vi "main 0.4.vi"() -> ()   [LabVIEW 2015]
uses:
  subvi/PHOIBOS/DEFINITIONS/DEF_dev_state.ctl
  subvi/PHOIBOS/DEFINITIONS/DEF_dev_type.ctl
  <vilib>/Utility/file.llb/Write Delimited Spreadsheet (DBL).vi
  subvi/Newport ESP301/Newport ESP301.lvlib
  subvi/sp_manip.llb/sp_manip_lib.lvlib
  subvi/sp_manip.llb/tcp_gateway.lvlib
panel:
  out "state":T1 items=["Off"=-1, "Standby"=0, "On"=1]
  in  "BasePath 2":path=path "Z:/PESdata"
  out "ESP_con?":bool caption="ESP301"
  out "phoib_con?":bool caption="PHOIBOS"
  out "manip_con?":bool caption="manipulator"
  out "cam_con?":bool caption="camera"
  in  "main_close":bool
  in  "Tab Control":enum32{"Live", "Measure", "Settings", "Devices"}(tab)
  in  "cam_dark#":u32 max=1000
  in  "cam_dark":bool
  out "cam_fps":dbl(slide)=8.239338102188393 caption="FPS" scale=0.1..50.0
  out "cam_burst_progress":u8(slide) scale=0.0..200.0
  in  "cam_burstnr":u32 max=1000
  in  "cam_burst":bool
  in  "ESP_delta":dbl
  in  "ESP_+ 2":bool
  in  "ESP_+":bool
  in  "ESP_go":bool
  in  "ESP_dest_t":dbl caption="Delay"
  in  "ESP_dest":dbl caption="Position"
  in  "ESP_set_t0":bool
  in  "phoib_I_6s":dbl=3200.0
  in  "phoib_I_5s":dbl=1400.0
  in  "phoib_I_4s":dbl=4.2
  in  "phoib_I_3s":dbl
  in  "phoib_I_2s":dbl=35.0
  in  "phoib_I_1s":dbl=21.9
  in  "phoib_standby":bool
  in  "phoib_set":bool
  out "phoib_I_6":dbl caption="Screen Voltage"
  out "phoib_I_5":dbl caption="Detctor Voltage"
  out "phoib_I_4":dbl caption="Work Function"
  out "phoib_I_3":dbl caption="Coil Current"
  out "phoib_I_2":dbl caption="Pass Energy"
  out "phoib_I_1":dbl caption="Kinetic Energy"
  out "CCD temp [°C]":i32=-12
  out "electronics temp [°C]":i32=30
  out "Saved Positions":string[][](table)=[["ertwertwert", "-2.299945", "-2.030214", "38.900024", "50.000762", "0.000887", "-97.998082"], ["uztgugt", "-14.999451", "-13.638894", "442.380066", "13.998380", "-1.893758", "-76.305838"], ["asdf", "-14.999451", "-13.638894", "442.380066", "13.998380", "-1.893758", "-76.305838"], ["test3", "-14.999451", "-13.638894", "441.380066", "13.998380", "-1.893758", "-76.305838"]]
  in  "Save Pos":bool
  in  "Load":bool
  in  "Delete":bool
  in  "ManipRel":dbl=1.0
  in  "ManipRel +":bool
  in  "ManipRel -":bool
  in  "manip.rel.select":enum32{"x", "y", "z", "polar", "tilt", "azimut"}(radio)=enum."polar"
  in  "Move Abs":bool
  in  "stop manip":bool
  in  "dest":dbl[](array[numeric])=[0.007141549166819264, -0.009888298846365134, 431.30615234375, 89.00040512814502, 1.109125024699864, -227.9162918846475] caption="destinations" format="%#.5g"
  out "names":string[](array[string])=["x", "y", "z", "polar", "tilt", "azimut"]
  out "pos":dbl[](array[numeric])=[0.007141549166819264, -0.009888298846365134, 431.30615234375, 89.00040512814502, 1.109125024699864, -227.9162918846475] caption="positions" format="%.5f"
  out "Intensity Graph":dbl[][](graph)
  in  "Exposure [ms]":u32=20
  in  "Mode":T2(ring)=enum."WideAngleMode"
  in  "VoltageRange":enum16{"3.5kV", "1.5kV", "400V", "100V", "10V"}(ring)=enum."400V"
  out "ESP_pos":dbl caption="Position"
  out "ESP_delay":dbl caption="Delay"
  in  "ESP_t0":dbl caption="Time Zero @"
  in  "binning":u16(ring)=2 items=["X 1", "X 2", "X 4", "X 8"]
  in  "Gain":bool
  out "max value":u16=55
  out "phoib_I_7":dbl caption="Conversion Voltage"
  in  "phoib_I_7s":dbl
  in  "phoib_I_8s":dbl
  in  "phoib_I_9s":dbl
  out "phoib_I_8":dbl caption="FD1"
  out "phoib_I_9":dbl caption="FD2"
  in  "cam_dark?":bool caption="subtract dark?"
  out "opti_frames":dbl=25.0 caption="#steps_opti"
  out "opti_current_frame":i32=25
  out "Measurement Progress":u8(slide) scale=0.0..100.0
  out "Camera Aquisition":u8(slide) scale=0.0..100.0
  in  "Optimize":bool
  in  "OptiStepSize":dbl=-1.0 caption="Step Size"
  in  "OptiRange":dbl=25.0 caption="Range"
  in  "meas_axis":string(combo)="tilt" caption="Axis"
  in  "meas_avg":i32=60 caption="Frames2Average"
  in  "OptiCancel":bool
  out "#steps_opti":dbl=25.0
  out "current_step_opti":i32=25
  out "ETA":string
  in  "BasePath":path=path "Z:/PESdata"
  in  "Path":path=path "Z:/software/ManipulatorControl/save.txt"
  in  "ROI Bottom":i32=32
  in  "ROI Top":i32=1
  in  "ROI Right":i32=40
  in  "ROI Left":i32=1
  in  "ESP Axis":i32=1 min=1 max=3
  in  "manip_init":bool
  in  "manip_release":bool
  in  "phoib_init":bool
  in  "phoib_release":bool
  in  "ESP_init":bool
  in  "ESP_release":bool
  in  "ESP301 VISA":refnum<visa-resource-name>="COM8"
  in  "cam_boardnr":i32
  in  "cam_init":bool
  in  "cam_release":bool
  out "error out":errorcluster
  out "error out 2":errorcluster
  # "step _ of _"
  # "step _ of _"
  # "manip"
  # "phoib"
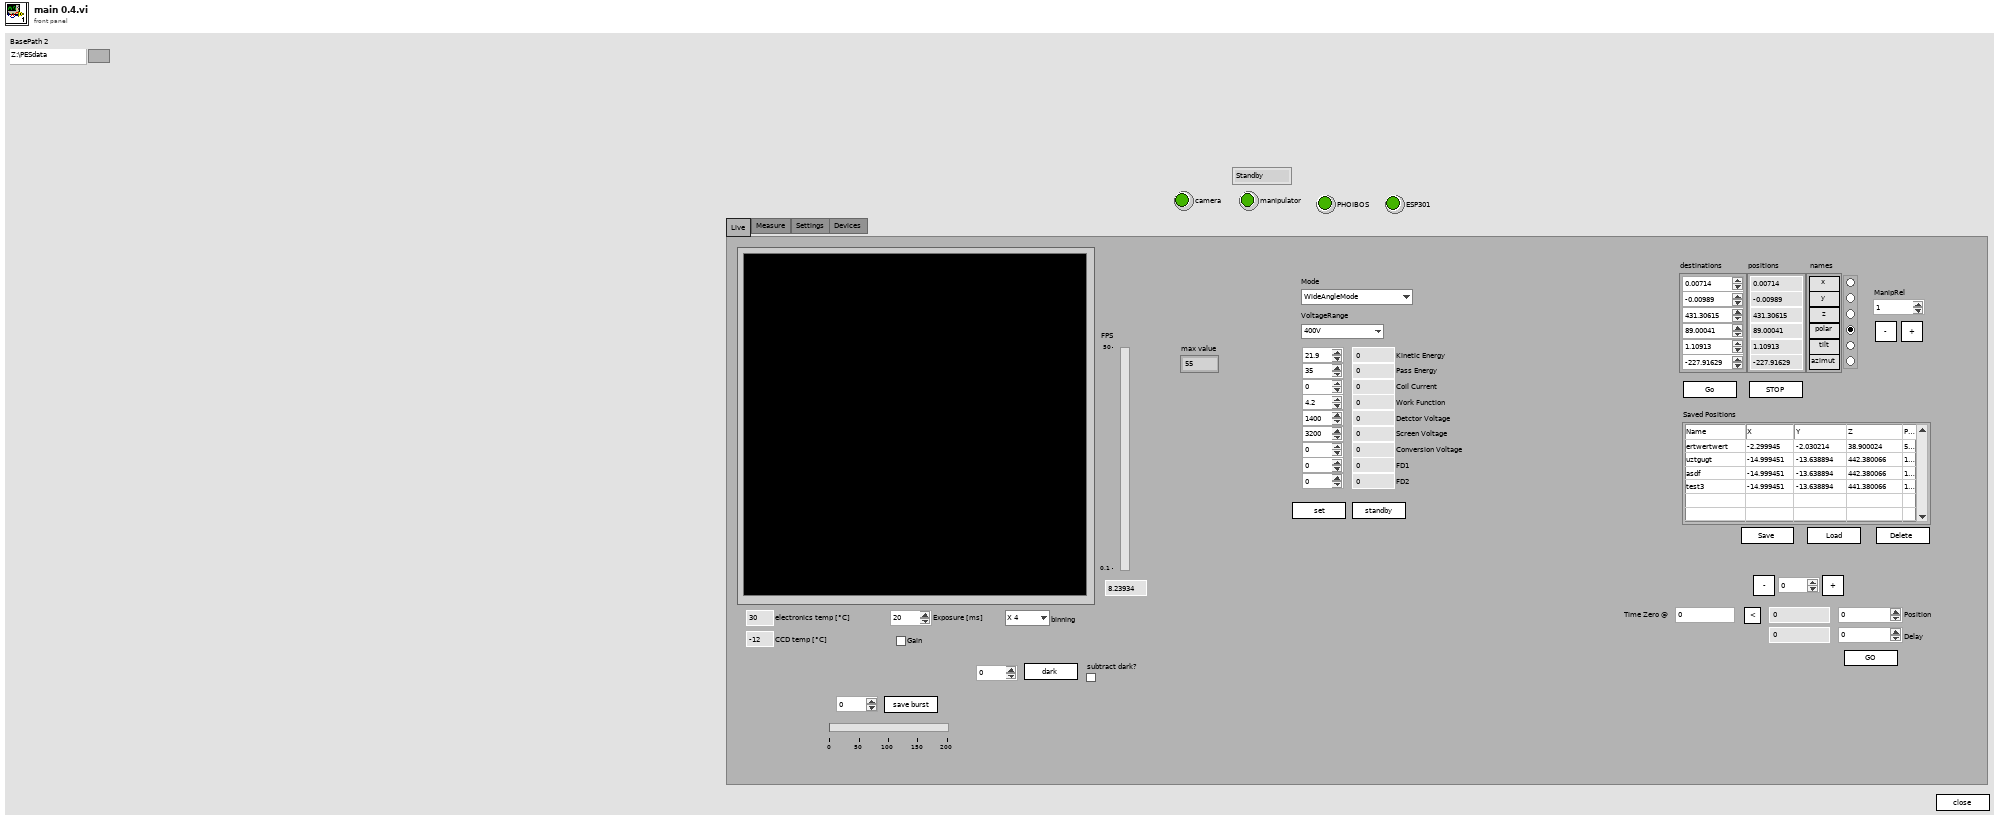
[diagram p1: front panel]
types:
  T1 = typedef "DEF_dev_state.ctl" = i32
  T2 = enum16{"HighMagnification", "MediumMagnification", "LowMagnification", "HighAngularDispersion", "MediumAngularDispersion", "LowAngularDispersion", "WideAngleMode", "LargeArea", "MediumArea", "SmallArea", "HighMagnification2", "SmallArea2", "ImagingMode"}
  T3 = cluster{"Camera type":u32, "Operating mode\nHP & QE / HS & DiCam Pro ":u32, "Frame trigger \n(High Performance and QE only)":u16, "Sequence trigger":u16, "Low Light\n(QE only)":bool, "Gain":bool, "Horzontal\nbinning":u16, "Vertical\nbinning ":u16, "ROI Left":i32, "ROI Right":i32, "ROI Top":i32, "ROI Bottom":i32}
  T4 = enum16{"open", "replace", "create", "open or create", "replace or create", "replace or create with confirmation"}
  T5 = cluster{"Axis_Name":string, "Axis_Type":string, "Axis_Position":dbl, "continous":bool, "moving":bool}[]
  T6 = cluster{"Axis_Name":string, "Axis_Type":string, "Axis_Position":dbl, "continous":bool, "moving":bool}
  T7 = typedef "DEF_dev_type.ctl" = enum32{"devA (analyzer)", "devD (detector)"}
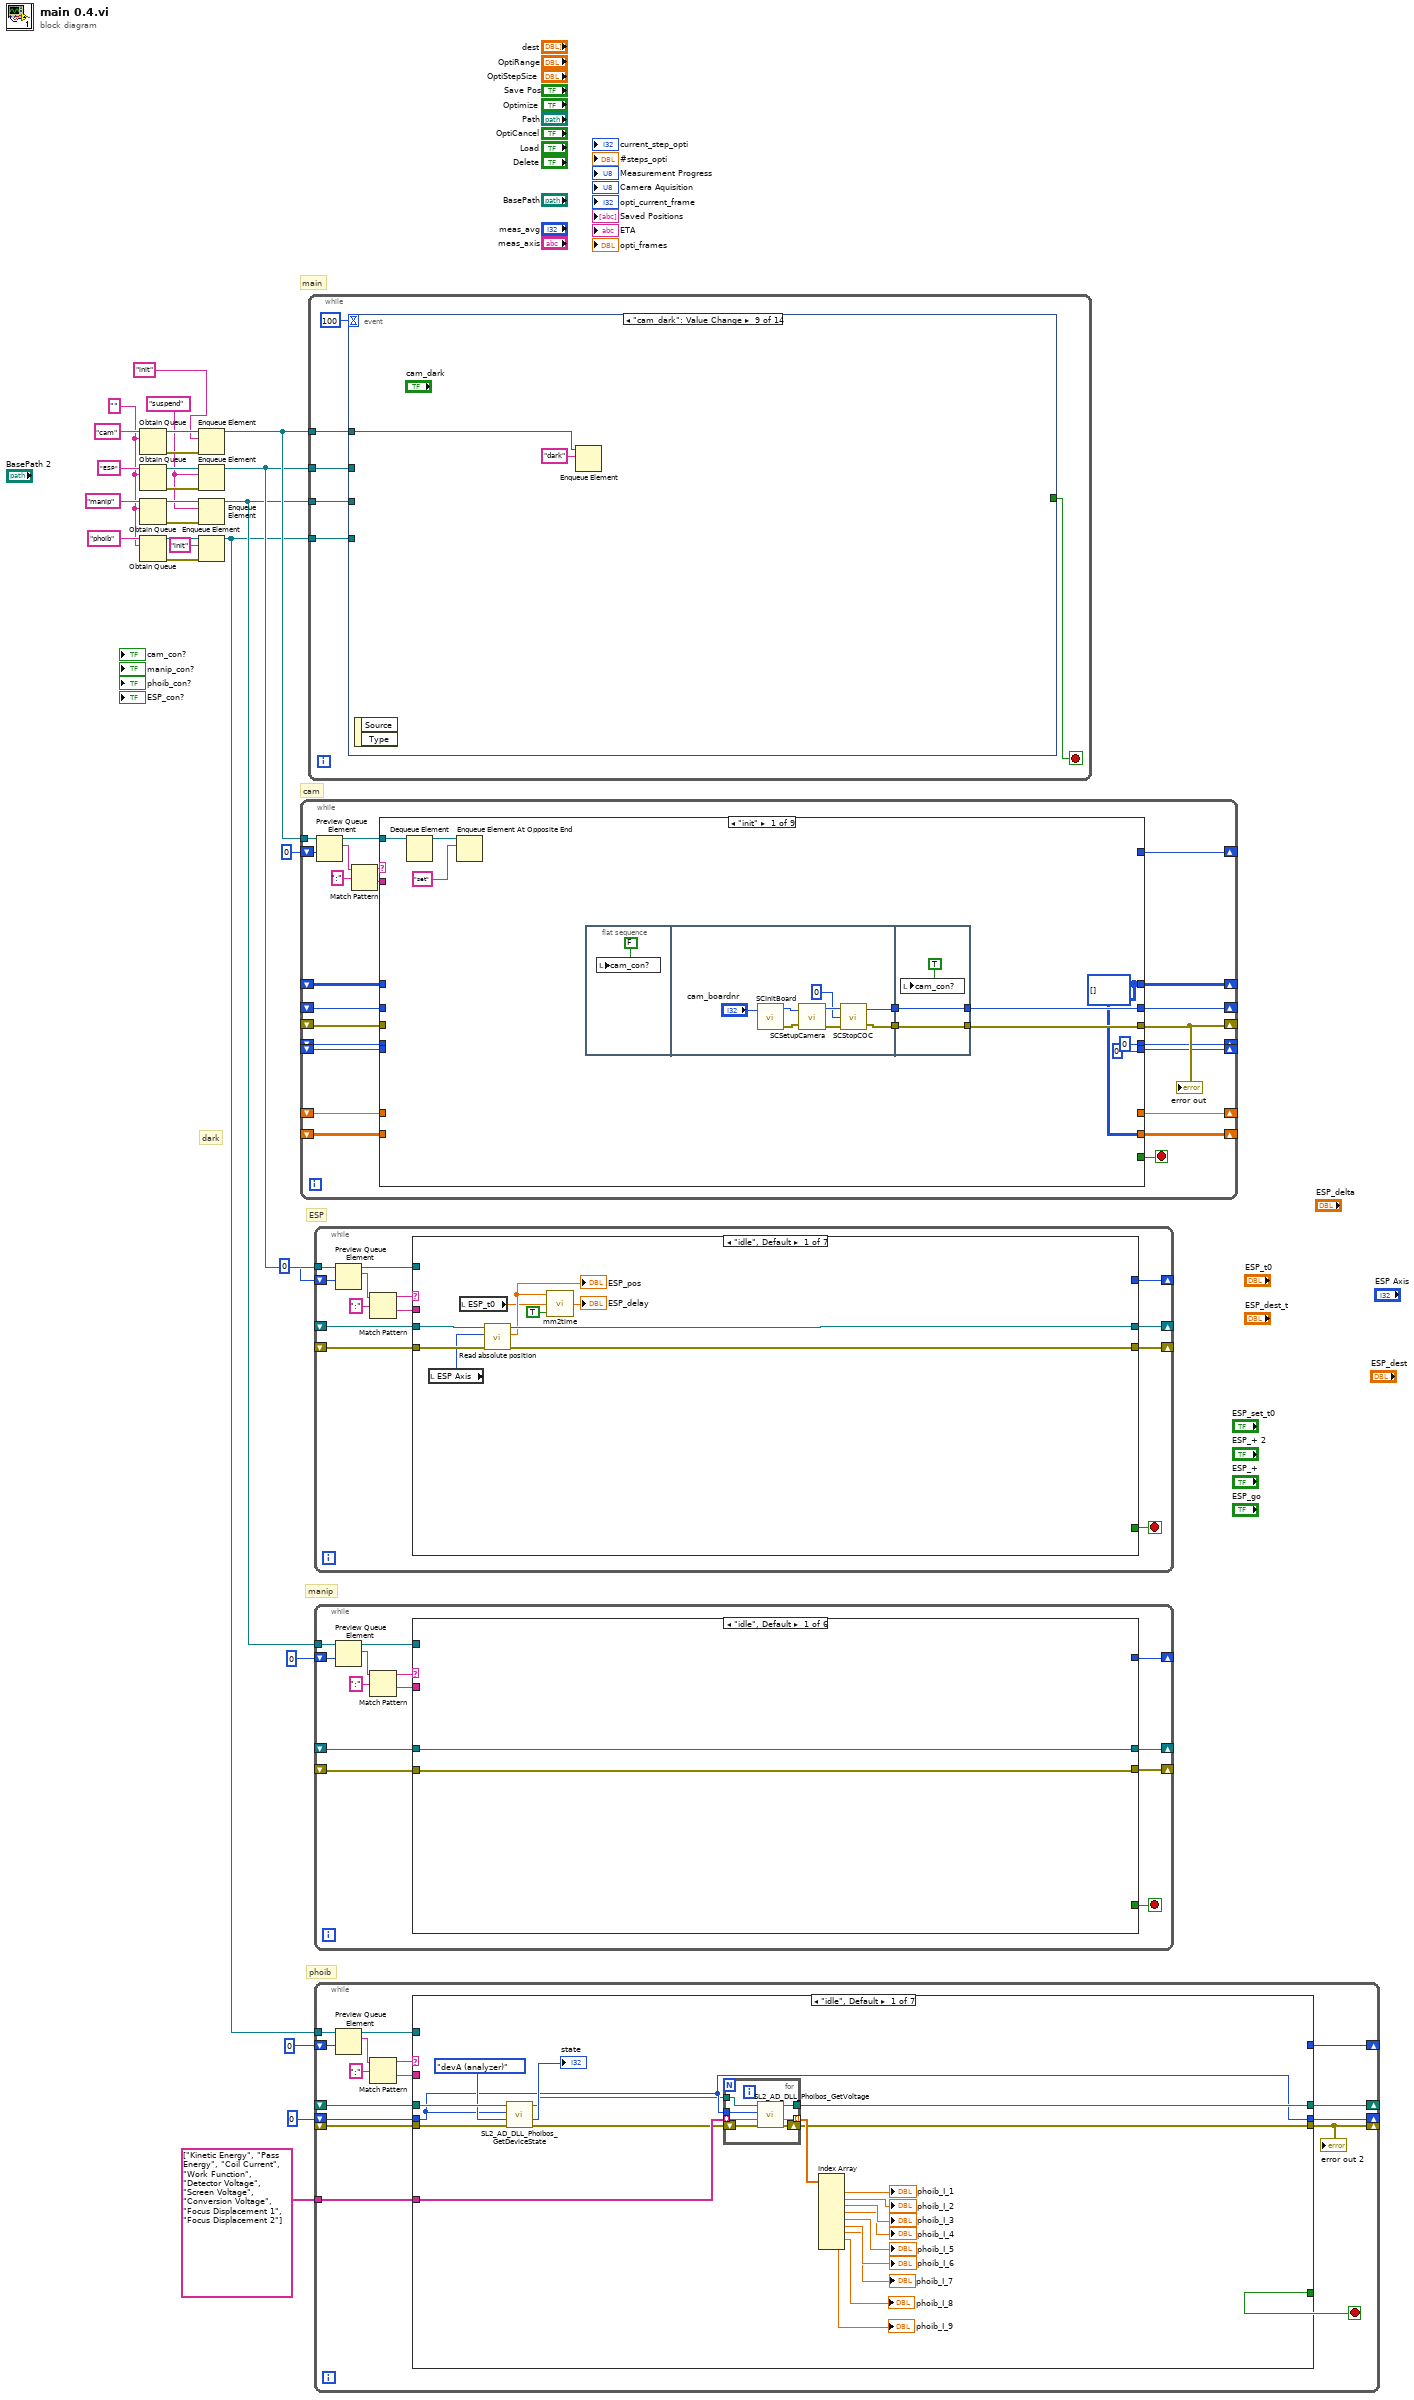
[diagram p0: block diagram]
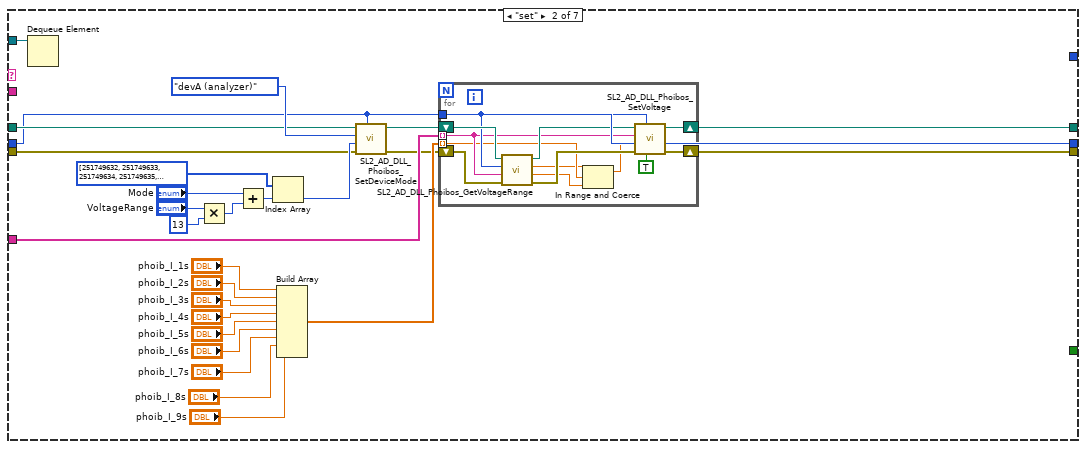
[diagram p2: hidden frame]
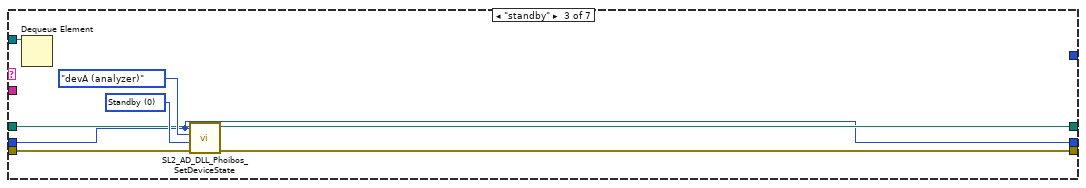
[diagram p3: hidden frame]
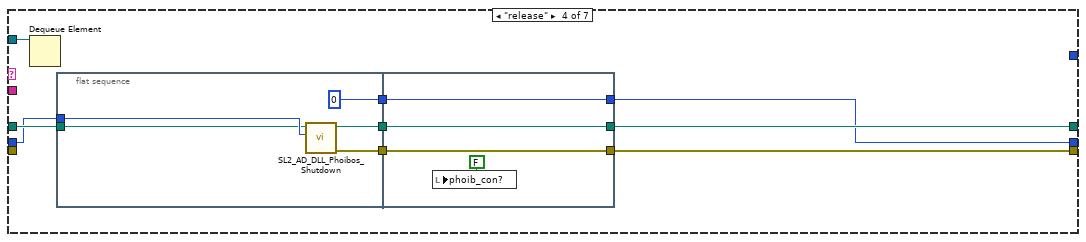
[diagram p4: hidden frame]
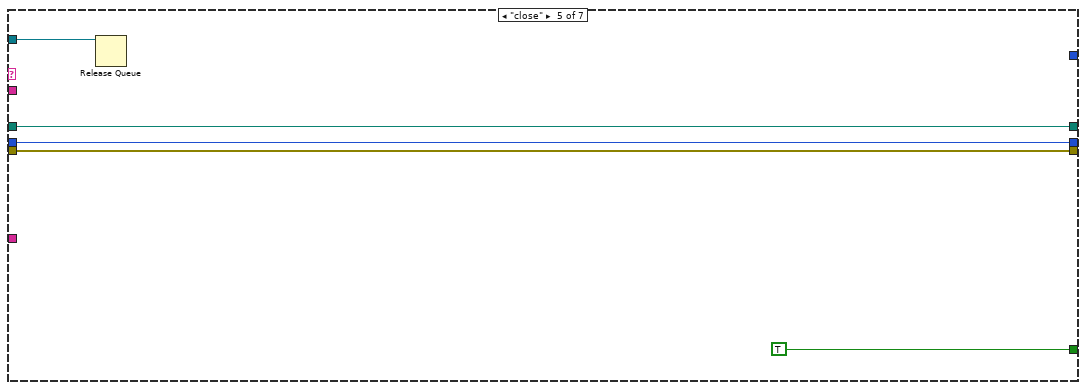
[diagram p5: hidden frame]
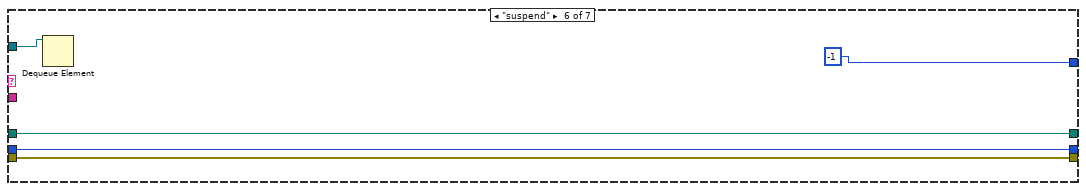
[diagram p6: hidden frame]
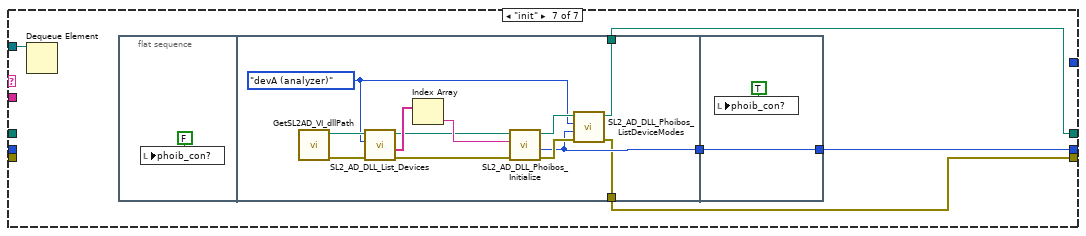
[diagram p7: hidden frame]
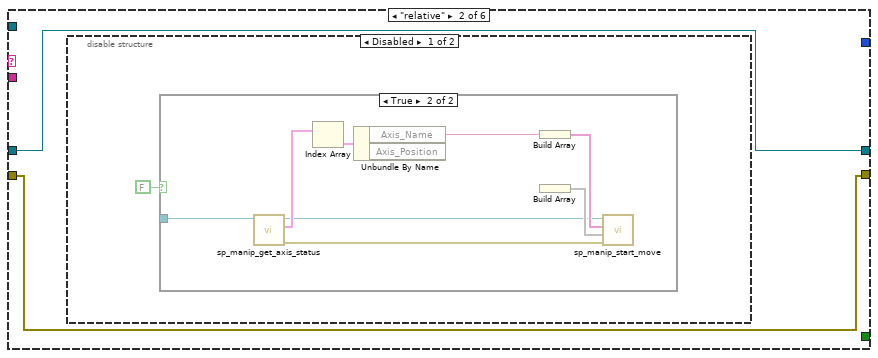
[diagram p8: hidden frame]
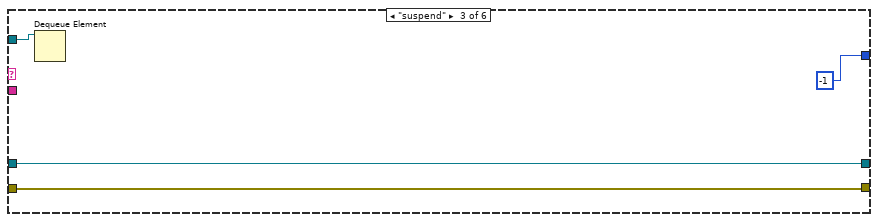
[diagram p11: hidden frame]
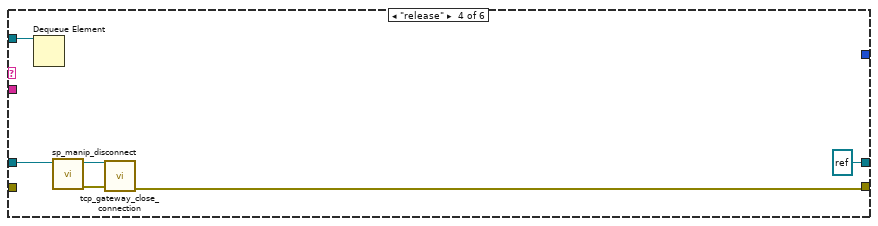
[diagram p12: hidden frame]
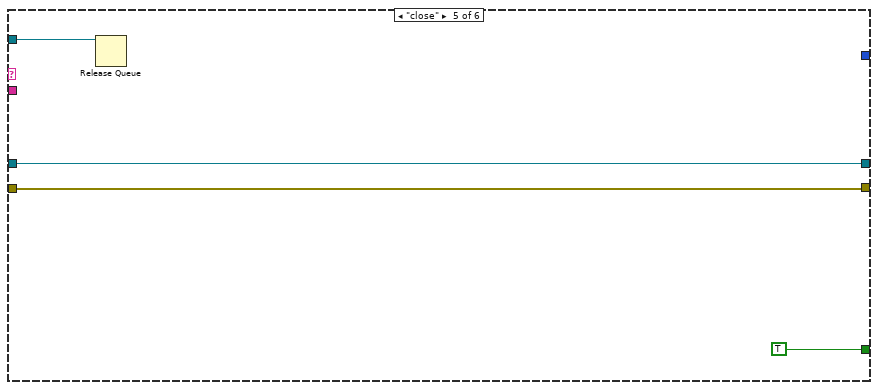
[diagram p13: hidden frame]
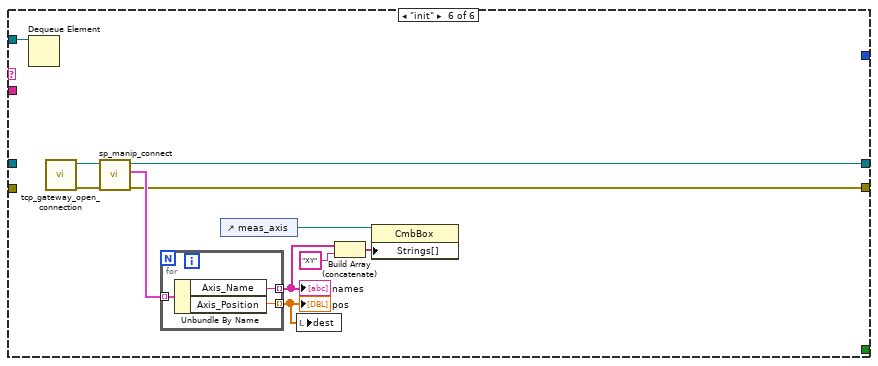
[diagram p14: hidden frame]
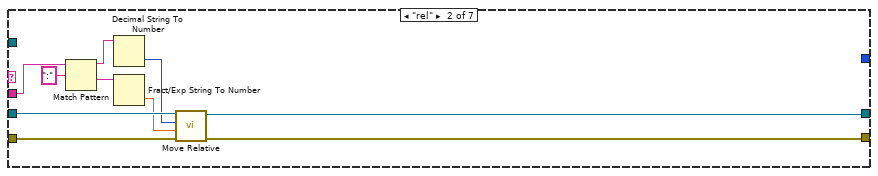
[diagram p15: hidden frame]
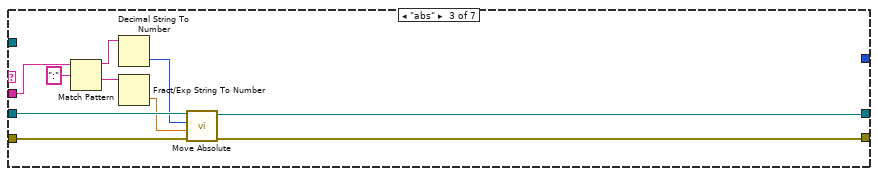
[diagram p16: hidden frame]
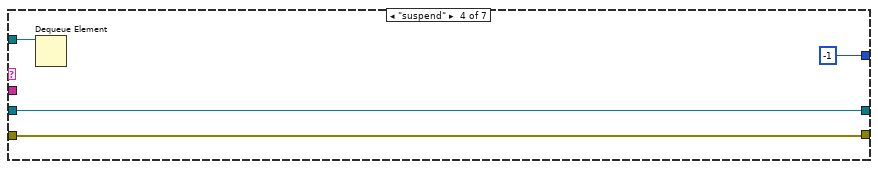
[diagram p17: hidden frame]
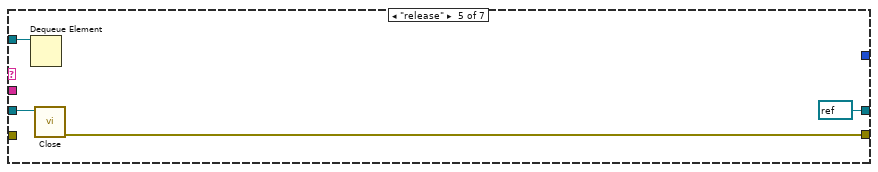
[diagram p18: hidden frame]
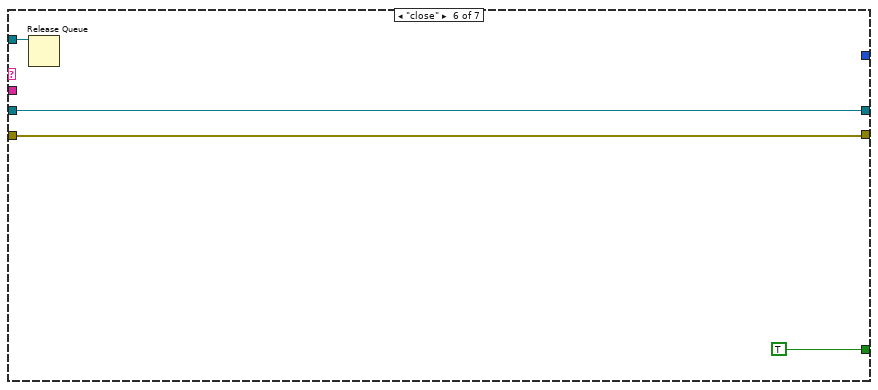
[diagram p19: hidden frame]
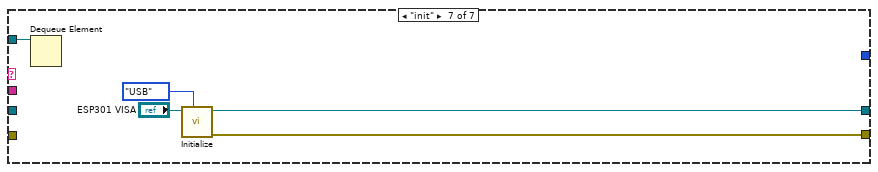
[diagram p20: hidden frame]
diagram:
  w13 = "suspend" ("name (unnamed)")
  w12 = "" ("name (unnamed)")
  # "dark"
  # "phoib"
  # "manip"
  # "ESP"
  # "cam"
  # "main"
  n1 = Obtain Queue(name (unnamed)="cam", element data type=w12) -> (queue out=w25:refnum<queue>, error out=w24:errorcluster)  [unwired: 3 in, 1 out]
  n2 = Obtain Queue(name (unnamed)="ESP", element data type=w12) -> (queue out=w21:refnum<queue>, error out=w22:errorcluster)  [unwired: 3 in, 1 out]
  n3 = Obtain Queue(name (unnamed)="manip", element data type=w12) -> (queue out=w18:refnum<queue>, error out=w17:errorcluster)  [unwired: 3 in, 1 out]
  n4 = Obtain Queue(name (unnamed)="phoib", element data type=w12) -> (queue out=w15:refnum<queue>, error out=w16:errorcluster)  [unwired: 3 in, 1 out]
  n5 = Enqueue Element(queue=w25, element="init" ("name (unnamed)"), error in (no error)=w24) -> (queue out=w23:refnum<queue>)  [unwired: 1 in, 2 out]
  n6 = Enqueue Element(queue=w21, element=w13, error in (no error)=w22) -> (queue out=w11:refnum<queue>)  [unwired: 1 in, 2 out]
  n7 = Enqueue Element(queue=w18, element=w13, error in (no error)=w17) -> (queue out=w10:refnum<queue>)  [unwired: 1 in, 2 out]
  n8 = Enqueue Element(queue=w15, element="init", error in (no error)=w16) -> (queue out=w9:refnum<queue>)  [unwired: 1 in, 2 out]
  n9 = while {
    tunnel: w23 -> [w49]
    shift-right: [w43] -> _
    shift-left: _ -> [w42]
    shift-right: [w41] -> _
    shift-left: _ -> [w37]
    shift-right: [w40] -> _
    shift-left: _ -> [w36]
    shift-right: [w39] -> _
    shift-left: _ -> [w35]
    shift-right: [w38] -> _
    shift-left: _ -> [w34]
    shift-right: [w31] -> _
    shift-left: 0 -> [w32]
    shift-right: [w30] -> _
    shift-left: _ -> [w29]
    shift-right: [w28] -> _
    shift-left: _ -> [w27]
    stop <- w33 stop-if-true
    n10 = Preview Queue Element(queue=w49, timeout in ms (-1)=w32) -> (queue out=w48:refnum<queue>, element=w47:string)  [unwired: 1 in, 2 out]
    n11 = Match Pattern(string=w47, regular expression=":") -> (before substring=w44:string, after substring=w45:string)  [unwired: 1 in, 2 out]
    n12 = case shown="\"init\"" w44 {
      tunnel: w48 -> [w58 w84 w127 w180 w192 _ w225 _ w285]
      tunnel: w45 -> [_ _ w140 _ _ _ _ w260 _]
      tunnel: [w50 w73 w137 w179 w190 w215 w230 w258 w283] -> w43
      tunnel: w42 -> [_ _ w137 w179 w190 w215 w230 w258 w283]
      tunnel: [w57 w85 w136 u64 0 ("Hout") w189 w206 w229 w257 w282] -> w41
      tunnel: [w59 w86 w133 w174 w188 w209 w228 w256 w281] -> w40
      tunnel: [0 ("Horizontal size") w77 w135 w178 w187 w214 w227 w255 w280] -> w39
      tunnel: [0 ("Vertical size") w76 w134 w177 w186 w213 w226 w254 w279] -> w38
      tunnel: w37 -> [_ w88 w136 w176 w189 w205 w231 w257 w282]
      tunnel: w36 -> [_ w87 w133 _ w188 w204 w228 w267 w281]
      tunnel: w35 -> [_ _ w135 w178 w187 w214 w227 w255 w280]
      tunnel: w34 -> [_ _ w134 w177 w186 w213 w226 w254 w279]
      tunnel: [_ _ _ _ TRUE _ _ _ _] -> w33
      tunnel: [_ _ _ _ _ _ _ _ -1] -> w31
      tunnel: [_ _ _ _ _ w201 _ _ _] -> w30
      tunnel: w29 -> [_ _ _ _ _ w200 _ _ _]
      tunnel: [w50 w72 w105 w172 w185 w195 w232 w253 w278] -> w28
      tunnel: w27 -> [_ w72 w105 w172 w185 w195 _ w253 w278]
      frame "init" {
        w50 = u16[][] []
        n13 = Dequeue Element(queue=w58) -> (queue out=w52:refnum<queue>)  [unwired: 2 in, 3 out]
        n14 = Enqueue Element At Opposite End(queue=w52, element="set") -> ()  [unwired: 2 in, 3 out]
        n15 = flat-sequence {
          tunnel: [w61] -> w56
          tunnel: [w62] -> w55
          tunnel: [w70] -> w57
          tunnel: [w71] -> w59
          tunnel: w56 -> [w71]
          tunnel: w55 -> [w70]
          frame #0 {
            n16 = local write "cam_con?"(FALSE ("cam_con?")) -> ()
          }
          frame #1 {
            n17 = call "SCInitBoard.vi"("boardnr"="cam_boardnr") -> ("Hout"=w65:u32, "error out"=w66:errorcluster)  [unwired: 1 in, 1 out]
            n18 = call "SCSetupCamera.vi"("Handle"=w65, "error in (no error)"=w66) -> ("Hout"=w67:u64, "error out"=w68:errorcluster)  [unwired: 1 out]
            n19 = call "SCStopCOC.vi"("error in (no error)"=w68, "Stop mode"=0, "Handle"=w67) -> ("error out"=w61:errorcluster, "Hout"=w62:u64)
          }
          frame #2 {
            n20 = local write "cam_con?"(TRUE ("cam_con?")) -> ()
          }
        }
      }
      frame "set" {
        w83 = u32 1 ("Operating mode\nHP & QE / HS & DiCam Pro")
        n21 = Dequeue Element(queue=w84) -> ()  [unwired: 2 in, 4 out]
        n22 = Bundle By Name(cluster=cluster{"Delay":dbl, "Exposure ":dbl} {"Delay"=0.0, "Exposure "=0.0} ("Delay and exposure"), "Exposure"="Exposure [ms]") -> (w80:cluster{"Delay":dbl, "Exposure ":dbl})
        n23 = Bundle By Name(cluster=T3 {"Camera type"=0, "Operating mode\nHP & QE / HS & DiCam Pro "=0, "Frame trigger \n(High Performance and QE only)"=0, "Sequence trigger"=0, "Low Light\n(QE only)"=FALSE, "Gain"=FALSE, "Horzontal\nbinning"=0, "Vertical\nbinning "=0, "ROI Left"=1, "ROI Right"=20, "ROI Top"=1, "ROI Bottom"=15} ("Camera controls"), "Operating mode\nHP & QE / HS & DiCam Pro"=w83, "Horzontal\nbinning"="binning", "Vertical\nbinning"="binning", "ROI Left"="ROI Left", "ROI Right"="ROI Right", "ROI Top"="ROI Top", "ROI Bottom"="ROI Bottom", "Gain"="Gain") -> (w99:T3)
        n24 = call "New delay and exposure forma.vi"("Operating mode\nHP & QE / HS & DiCam Pro"=w83, "Delay and exposure"=w80) -> ("Output table"=w100:string)  [unwired: 3 in]
        n25 = call "SCStopCOC.vi"("error in (no error)"=w87, "Stop mode"=0, "Handle"=w88) -> ("error out"=w104:errorcluster, "Hout"=w103:u64)
        n26 = call "SCSetCoC.vi"("error in (no error)"=w104, "Delay and exposure table"=w100, "Camera controls"=w99, "Handle"=w103) -> ("error out"=w92:errorcluster, "Hout"=w91:u64)  [unwired: 1 out]
        n27 = call "SCGetImageSize.vi"("Handle"=w91, "error in (no error)"=w92) -> ("Hout"=w90:u64, "error out"=w89:errorcluster, "Horizontal size"=w77:i32, "Vertical size"=w76:i32)  [unwired: 2 out]
        n28 = Greater?(x=w77, y=w76) -> (0:w78:bool)
        n29 = Select(t=w77, s=w78, f=w76) -> (s? t:f=w75:i32)
        n30 = Initialize Array(u16 0 ("dimension size"), w76, w77) -> (w73:u16[][])
        n31 = call "SCRun.vi"("error in (no error)"=w89, "Run mode"=0, "Handle"=w90) -> ("error out"=w86:errorcluster, "Hout"=w85:u64)  [unwired: 1 out]
        n32 = property on="Intensity Graph" class="IntGraph (strict)"("XScale.Maximum"=w75, "YScale.Maximum"=w75) -> ()  [unwired: 2 in, 2 out]
      }
      frame "burst" {
        w107 = "\r"
        w108 = "\t"
        n33 = local read "Exposure [ms]"() -> (w116:u32)
        n34 = local read "binning"() -> (w118:u16)
        n35 = Dequeue Element(queue=w127) -> ()  [unwired: 2 in, 4 out]
        n36 = local read "Gain"() -> (w117:bool)
        n37 = Boolean To (0,1)(Boolean=w117) -> (0, 1=w119:i16)
        n38 = Get Date/Time In Seconds() -> (seconds since 1Jan1904=w132:timestamp)
        n39 = Match Pattern(string=w140, regular expression=":") -> (before substring=w139:string, after substring=w138:string)  [unwired: 1 in, 2 out]
        n40 = Number To Decimal String(number=w116) -> (decimal integer string=w121:string)  [unwired: 1 in]
        n41 = Number To Decimal String(number=w119) -> (decimal integer string=w123:string)  [unwired: 1 in]
        n42 = Number To Decimal String(number=w118) -> (decimal integer string=w125:string)  [unwired: 1 in]
        n43 = String To Path(string=w138) -> (path=w130:path)
        n44 = Format Date/Time String(time format string (%c)="%Y.%m.%d-%H.%M.%S", seconds (now)=w132) -> (date/time string=w129:string)  [unwired: 1 in]
        n45 = Build Path(base path=w130, name or relative path=w129) -> (appended path=w128:path)
        n46 = Decimal String To Number(string=w139) -> (number=w106:i32)  [unwired: 2 in, 1 out]
        n47 = Create Folder(path (use dialog)=w128) -> (created path=w111:path)  [unwired: 2 in, 2 out]
        n48 = Concatenate Strings("Exposure:", w108, w121, w107, "Gain:", w108, w123, w107, "binning", w108, w125, w107) -> (w115:string)
        n49 = Build Path(base path=w111, name or relative path="info.txt") -> (appended path=w110:path)
        n50 = Open/Create/Replace File(file path (use dialog)=w110, operation (0:open)=T4."replace or create") -> (refnum out=w113:refnum<file>)  [unwired: 4 in, 2 out]
        n51 = Write to Text File(file (use dialog)=w113, text=w115) -> (refnum out=w114:refnum<file>)  [unwired: 2 in, 2 out]
        n52 = Close File(refnum=w114) -> ()  [unwired: 1 in, 2 out]
        n53 = for {
          N: w106 -> [_]
          tunnel: w137 -> [w161]
          tunnel: w136 -> [w158]
          tunnel: w133 -> [w157]
          tunnel: w135 -> [w160]
          tunnel: w134 -> [w159]
          tunnel: w111 -> [w153]
          tunnel: 1000 ("x") -> [w151]
          tunnel: w105 -> [w144]
          i -> [w146]
          w162 = 0 items=["Normal", "Upside down"] ("mode")
          n54 = while {
            tunnel: [w170] -> w155
            tunnel: [w169] -> w156
            tunnel: w158 -> [w168]
            tunnel: w157 -> [w167]
            stop <- w171 stop-if-true
            n55 = call "SCWaitForImage.vi"("Handle"=w168, "error in (no error)"=w167) -> ("Hout"=w169:u64, "Image Valid"=w171:bool, "error out"=w170:errorcluster)  [unwired: 15 in]
          }
          n56 = Add(x=w151, y=w146) -> (x+y=w150:i32)
          n57 = Number To Decimal String(number=w150) -> (decimal integer string=w149:string)  [unwired: 1 in]
          n58 = String Subset(string=w149, offset (0)=1) -> (substring=w147:string)  [unwired: 1 in]
          n59 = local read "cam_dark?"() -> (w142:bool)
          n60 = Build Path(base path=w153, name or relative path=w147) -> (appended path=w152:path)
          n61 = call "SCGet12BitImage.vi"("mode"=w162, "Input array"=w161, "error in (no error)"=w155, "Vertical size"=w159, "Horizontal size"=w160, "Handle"=w156) -> ("error out"=w154:errorcluster, "imgdata"=w145:u16[][])  [unwired: 1 in, 1 out]
          n62 = case shown="False" w142 {
            tunnel: w145 -> [w163 w166]
            tunnel: w144 -> [_ w165]
            tunnel: [w163 w164] -> w143
            frame False {
            }
            frame True {
              n63 = Subtract(x=w166, y=w165) -> (x-y=w164:dbl[][])
            }
          }
          n64 = call-poly <vilib>:"Write Delimited Spreadsheet.vi"("file path (dialog if empty)"=w152, "2D data"=w143, "error in (no error)"=w154) -> ()  [unwired: 11 in, 2 out]
          n65 = local write "Intensity Graph"(w143) -> ()
          "cam_burst_progress" <- w146
        }
        n66 = property on="cam_burst_progress" class="Slide (strict)"("Scale.Maximum"=w106) -> ()  [unwired: 2 in, 2 out]
      }
      frame "release" {
        n67 = Dequeue Element(queue=w180) -> ()  [unwired: 2 in, 4 out]
        n68 = flat-sequence {
          tunnel: w176 -> [w182]
          tunnel: [w181] -> w173
          tunnel: [w184] -> w174
          tunnel: w173 -> [w184]
          frame #0 {
            n69 = call "SCCloseBoard.vi"("Handle"=w182) -> ("error out"=w181:errorcluster)  [unwired: 1 in, 2 out]
          }
          frame #1 {
            n70 = local write "cam_con?"(FALSE ("cam_con?")) -> ()
          }
        }
      }
      frame "close" {
        n71 = Release Queue(queue=w192) -> ()  [unwired: 2 in, 3 out]
      }
      frame "idle", Default {
        w212 = 0 items=["Normal", "Upside down"] ("mode")
        n72 = while {
          tunnel: [w223] -> w202
          tunnel: [w222] -> w203
          tunnel: w205 -> [w221]
          tunnel: w204 -> [w220]
          stop <- w224 stop-if-true
          n73 = call "SCWaitForImage.vi"("Handle"=w221, "error in (no error)"=w220) -> ("Hout"=w222:u64, "Image Valid"=w224:bool, "error out"=w223:errorcluster)  [unwired: 15 in]
        }
        n74 = call "SCGet12BitImage.vi"("mode"=w212, "Input array"=w215, "error in (no error)"=w202, "Vertical size"=w213, "Horizontal size"=w214, "Handle"=w203) -> ("error out"=w210:errorcluster, "imgdata"=w196:u16[][], "Hout"=w211:u64)  [unwired: 1 in]
        n75 = case shown="False" "cam_dark?" {
          tunnel: w196 -> [w216 w219]
          tunnel: w195 -> [_ w218]
          tunnel: [w216 w217] -> w194
          frame False {
          }
          frame True {
            n76 = Subtract(x=w219, y=w218) -> (x-y=w217:dbl[][])
          }
        }
        "Intensity Graph" <- w194
        n77 = Array Max & Min(array=w194) -> (max value=→"max value":dbl)  [unwired: 3 out]
        n78 = call "SCGetStatus.vi"("Handle"=w211, "error in (no error)"=w210) -> ("Hout"=w206:u64, "Electronics temperature"=→"electronics temp [°C]":i32, "CCD temperature"=→"CCD temp [°C]":i32, "error out"=w209:errorcluster)  [unwired: 2 out]
        n79 = call <vilib>:"High Resolution Relative Seconds.vi"() -> ("relative seconds"=w201:dbl)
        n80 = Subtract(x=w201, y=w200) -> (x-y=w199:dbl)
        n81 = Reciprocal(x=w199) -> (1/x=→"cam_fps":dbl)
      }
      frame "dark" {
        n82 = Dequeue Element(queue=w225) -> ()  [unwired: 2 in, 4 out]
        n83 = Initialize Array(0.0, w226, w227) -> (w235:dbl[][])
        n84 = for {
          N: "cam_dark#" -> [_]
          tunnel: w227 -> [w246]
          tunnel: w226 -> [w245]
          tunnel: w230 -> [w243]
          shift-right: [w240] -> w234
          shift-left: w235 -> [w241]
          tunnel: w231 -> [w239]
          tunnel: w228 -> [w238]
          tunnel: [w237] -> w229
          n85 = while {
            tunnel: [w251] -> w244
            tunnel: [w250] -> w247
            tunnel: w239 -> [w249]
            tunnel: w238 -> [w248]
            stop <- w252 stop-if-true
            n86 = call "SCWaitForImage.vi"("Handle"=w249, "error in (no error)"=w248) -> ("Hout"=w250:u64, "Image Valid"=w252:bool, "error out"=w251:errorcluster)  [unwired: 15 in]
          }
          n87 = call "SCGet12BitImage.vi"("Input array"=w243, "error in (no error)"=w244, "Vertical size"=w245, "Horizontal size"=w246, "Handle"=w247) -> ("imgdata"=w242:u16[][], "Hout"=w237:u64)  [unwired: 2 in, 1 out]
          n88 = Add(x=w242, y=w241) -> (x+y=w240:dbl[][])
        }
        n89 = Divide(x=w234, y="cam_dark#") -> (x/y=w232:dbl[][])
      }
      frame "snap" {
        n90 = local read "BasePath 2"() -> (w269:path)
        n91 = local read "meas_avg"() -> (w264:i32)
        n92 = Initialize Array(u32 0 ("element"), w255, w254) -> (w266:u32[][])
        n93 = Build Path(base path=w269, name or relative path=w260) -> (appended path=w259:path)
        n94 = for {
          N: w264 -> [_]
          tunnel: w255 -> [w277]
          tunnel: w254 -> [w276]
          tunnel: w258 -> [w274]
          shift-right: [w271] -> w265
          shift-left: w266 -> [w273]
          shift-right: [w270] -> w256
          shift-left: w267 -> [w275]
          n95 = call "SCGet12BitImage.vi"("Input array"=w274, "error in (no error)"=w275, "Vertical size"=w276, "Horizontal size"=w277) -> ("error out"=w270:errorcluster, "imgdata"=w272:u16[][])  [unwired: 3 in, 1 out]
          n96 = Add(x=w272, y=w273) -> (x+y=w271:u32[][])
        }
        n97 = Divide(x=w265, y=w264) -> (x/y=w263:dbl[][])
        n98 = call-poly <vilib>:"Write Delimited Spreadsheet.vi"("file path (dialog if empty)"=w259, "format (%.3f)"="%d", "2D data"=w263, "transpose? (F)"=TRUE) -> ()  [unwired: 10 in, 2 out]
      }
      frame "suspend" {
        n99 = Dequeue Element(queue=w285) -> ()  [unwired: 2 in, 4 out]
      }
    }
    "error out" <- w40
  }
  n100 = while {
    tunnel: w23 -> [w289]
    tunnel: w11 -> [w288]
    tunnel: w10 -> [w287]
    tunnel: w9 -> [w286]
    stop <- w291 stop-if-true
    n101 = event shown="[8] \"cam_dark\": Value Change" {
      selector: _ -> [_ _ _ _ _ _ _ _ _ _ _ _ _ _]
      dyn-events: _ -> [_ _ _ _ _ _ _ _ _ _ _ _ _ _]
      timeout: 100 -> [_ _ _ _ _ _ _ _ _ _ _ _ _ _]
      tunnel: [_ TRUE _ _ _ _ _ _ _ _ _ _ _ _] -> w291
      tunnel: w289 -> [_ w301 w304 _ _ _ _ _ w330 w332 w333 _ _ _]
      tunnel: w288 -> [_ w300 _ w308 _ _ _ _ _ _ _ _ _ _]
      tunnel: w287 -> [_ w299 _ _ w314 _ _ _ _ _ _ _ _ _]
      tunnel: w286 -> [_ w298 _ _ _ w320 w326 w327 _ _ _ _ _ _]
      event Timeout {
        n102 = event-data() -> ()  [unwired: 1 in, 1 out]
      }
      event "main_close": Value Change {
        w292 = "close" ("element")
        w297 = "release" ("element")
        n103 = event-data() -> ()  [unwired: 1 in, 1 out]
        n104 = Enqueue Element(queue=w301, element=w297) -> (queue out=w296:refnum<queue>)  [unwired: 2 in, 2 out]
        n105 = Enqueue Element(queue=w300, element=w297) -> (queue out=w295:refnum<queue>)  [unwired: 2 in, 2 out]
        n106 = Enqueue Element(queue=w299, element=w297) -> (queue out=w294:refnum<queue>)  [unwired: 2 in, 2 out]
        n107 = Enqueue Element(queue=w298, element=w297) -> (queue out=w293:refnum<queue>)  [unwired: 2 in, 2 out]
        n108 = Enqueue Element(queue=w296, element=w292) -> ()  [unwired: 2 in, 3 out]
        n109 = Enqueue Element(queue=w295, element=w292) -> ()  [unwired: 2 in, 3 out]
        n110 = Enqueue Element(queue=w294, element=w292) -> ()  [unwired: 2 in, 3 out]
        n111 = Enqueue Element(queue=w293, element=w292) -> ()  [unwired: 2 in, 3 out]
      }
      event "cam_release", "cam_init": Value Change {
        n112 = event-data() -> ()  [unwired: 1 in, 2 out]
        n113 = Select(t="init" ("name (unnamed)"), s="cam_init", f="release" ("name (unnamed)")) -> (s? t:f=w303:string)
        n114 = Enqueue Element(queue=w304, element=w303) -> ()  [unwired: 2 in, 3 out]
      }
      event "ESP_release", "ESP_init": Value Change {
        n115 = event-data() -> ()  [unwired: 1 in, 2 out]
        n116 = Select(t="init" ("name (unnamed)"), s="ESP_init", f="release" ("name (unnamed)")) -> (s? t:f=w312:string)
        n117 = Enqueue Element(queue=w308, element=w312) -> ()  [unwired: 2 in, 3 out]
      }
      event "manip_init", "manip_release": Value Change {
        n118 = event-data() -> ()  [unwired: 1 in, 2 out]
        n119 = Flush Queue(queue=w314) -> (queue out=w313:refnum<queue>)  [unwired: 1 in, 2 out]
        n120 = Select(t="init" ("name (unnamed)"), s="manip_init", f="release" ("name (unnamed)")) -> (s? t:f=w316:string)
        n121 = Enqueue Element(queue=w313, element=w316) -> ()  [unwired: 2 in, 3 out]
      }
      event "phoib_release", "phoib_init": Value Change {
        n122 = event-data() -> ()  [unwired: 1 in, 2 out]
        n123 = Flush Queue(queue=w320) -> (queue out=w319:refnum<queue>)  [unwired: 1 in, 2 out]
        n124 = Select(t="init" ("name (unnamed)"), s="phoib_init", f="release" ("name (unnamed)")) -> (s? t:f=w322:string)
        n125 = Enqueue Element(queue=w319, element=w322) -> ()  [unwired: 2 in, 3 out]
      }
      event "phoib_standby": Value Change {
        n126 = event-data() -> ()  [unwired: 1 in, 2 out]
        n127 = Enqueue Element(queue=w326, element="standby") -> ()  [unwired: 2 in, 3 out]
      }
      event "phoib_set": Value Change {
        n128 = event-data() -> ()  [unwired: 1 in, 2 out]
        n129 = Enqueue Element(queue=w327, element="set") -> ()  [unwired: 2 in, 3 out]
      }
      event "cam_dark": Value Change {
        n130 = event-data() -> ()  [unwired: 1 in, 2 out]
        n131 = Enqueue Element(queue=w330, element="dark") -> ()  [unwired: 2 in, 3 out]
      }
      event "ROI Left", "ROI Right", "ROI Top", "ROI Bottom", "Exposure [ms]", "binning", "Gain": Value Change {
        n132 = event-data() -> ()  [unwired: 1 in, 6 out]
        n133 = Enqueue Element(queue=w332, element="set") -> ()  [unwired: 2 in, 3 out]
      }
      event "cam_burst": Value Change {
        n134 = event-data() -> ()  [unwired: 1 in, 1 out]
        n135 = local read "BasePath"() -> (w337:path)
        n136 = call "File Dialog"("start path"=w337) -> ("selected path"=w335:path, "cancelled"=w336:bool, "error out"=w334:errorcluster)  [unwired: 11 in, 1 out]
        n137 = case shown="False" w336 {
          tunnel: w335 -> [w340 _]
          tunnel: w334 -> [_ _]
          tunnel: w333 -> [w345 _]
          frame False {
            n138 = Path To String(path=w340) -> (string=w339:string)
            n139 = Number To Decimal String(number="cam_burstnr") -> (decimal integer string=w342:string)  [unwired: 1 in]
            n140 = Concatenate Strings("burst:" ("string"), w342, ":" ("string"), w339) -> (w338:string)
            n141 = Enqueue Element(queue=w345, element=w338) -> ()  [unwired: 2 in, 3 out]
          }
          frame True {
          }
        }
      }
      event "Move Abs": Value Change {
        n142 = event-data() -> ()  [unwired: 1 in, 1 out]
      }
      event "ManipRel +", "ManipRel -": Value Change {
        n143 = event-data() -> ()  [unwired: 1 in, 2 out]
        n144 = Negate(x="ManipRel") -> (-x=w347:dbl)
        n145 = Select(t=w347, s="ManipRel -", f="ManipRel") -> ()  [unwired: 1 out]
      }
      event "stop manip": Value Change {
        n146 = event-data() -> ()  [unwired: 1 in, 1 out]
      }
    }
  }
  n147 = while {
    tunnel: w11 -> [w356]
    shift-right: [w354] -> _
    shift-left: _ -> [w352]
    shift-right: [w353] -> _
    shift-left: _ -> [w351]
    shift-right: [w349] -> _
    shift-left: 0 -> [w350]
    stop <- w355 stop-if-true
    n148 = Preview Queue Element(queue=w356, timeout in ms (-1)=w350) -> (queue out=w359:refnum<queue>, element=w360:string)  [unwired: 1 in, 2 out]
    n149 = Match Pattern(string=w360, regular expression=":") -> (before substring=w358:string, after substring=w357:string)  [unwired: 1 in, 2 out]
    n150 = case shown="\"idle\", Default" w358 {
      tunnel: w359 -> [_ _ _ w394 w395 w402 w407]
      tunnel: w357 -> [_ w375 w387 _ _ _ _]
      tunnel: [_ _ _ _ _ TRUE _] -> w355
      tunnel: [w368 w377 w383 w392 refnum<visa-resource-name> refnum ("VISA resource name out") w399 w404] -> w354
      tunnel: [w367 w378 w384 w391 w397 w400 w403] -> w353
      tunnel: w352 -> [w370 w380 w385 w392 w398 w399 _]
      tunnel: w351 -> [w369 w379 w386 w391 _ w400 _]
      tunnel: [_ _ _ -1 _ _ _] -> w349
      frame "idle", Default {
        n151 = local read "ESP Axis"() -> (w362:i32)
        n152 = local read "ESP_t0"() -> (w365:dbl)
        n153 = call "Read absolute position.vi"("error in (no error)"=w369, "Axis (1)"=w362, "VISA resource name"=w370) -> ("error out"=w367:errorcluster, "Position (units)"=w366:dbl, "VISA resource name out"=w368:refnum<visa-resource-name>)  [unwired: 2 in]
        "ESP_pos" <- w366
        n154 = call "mm2time.vi"("fs?"=TRUE, "Offset (mm)"=w365, "distance (mm)"=w366) -> ("time in fs/ps seconds"=→"ESP_delay":dbl)
      }
      frame "rel" {
        n155 = Match Pattern(string=w375, regular expression=":") -> (before substring=w374:string, after substring=w373:string)  [unwired: 1 in, 2 out]
        n156 = Decimal String To Number(string=w374) -> (number=w372:i32)  [unwired: 2 in, 1 out]
        n157 = Fract/Exp String To Number(string=w373) -> (number=w371:dbl)  [unwired: 3 in, 1 out]
        n158 = call "Move Relative.vi"("error in (no error)"=w379, "Position (0 units)"=w371, "Axis (1)"=w372, "VISA resource name"=w380) -> ("error out"=w378:errorcluster, "VISA resource name out"=w377:refnum<visa-resource-name>)  [unwired: 2 in]
      }
      frame "abs" {
        n159 = Match Pattern(string=w387, regular expression=":") -> (before substring=w389:string, after substring=w388:string)  [unwired: 1 in, 2 out]
        n160 = Decimal String To Number(string=w389) -> (number=w382:i32)  [unwired: 2 in, 1 out]
        n161 = Fract/Exp String To Number(string=w388) -> (number=w381:dbl)  [unwired: 3 in, 1 out]
        n162 = call "Move Absolute.vi"("error in (no error)"=w386, "Position (0 units)"=w381, "Axis (1)"=w382, "VISA resource name"=w385) -> ("error out"=w384:errorcluster, "VISA resource name out"=w383:refnum<visa-resource-name>)  [unwired: 2 in]
      }
      frame "suspend" {
        n163 = Dequeue Element(queue=w394) -> ()  [unwired: 2 in, 4 out]
      }
      frame "release" {
        n164 = Dequeue Element(queue=w395) -> ()  [unwired: 2 in, 4 out]
        n165 = call "Close.vi"("VISA resource name"=w398) -> ("error out"=w397:errorcluster)  [unwired: 10 in]
      }
      frame "close" {
        n166 = Release Queue(queue=w402) -> ()  [unwired: 2 in, 3 out]
      }
      frame "init" {
        n167 = Dequeue Element(queue=w407) -> ()  [unwired: 2 in, 4 out]
        n168 = call "Initialize.vi"("VISA resource name"="ESP301 VISA", "Serial Link (RS232)"=enum16{"RS232", "USB"}."USB") -> ("VISA resource name out"=w404:refnum<visa-resource-name>, "error out"=w403:errorcluster)  [unwired: 7 in]
      }
    }
  }
  n169 = while {
    tunnel: w10 -> [w415]
    shift-right: [w413] -> _
    shift-left: _ -> [w411]
    shift-right: [w412] -> _
    shift-left: _ -> [w410]
    shift-right: [w408] -> _
    shift-left: 0 -> [w409]
    stop <- w414 stop-if-true
    n170 = Preview Queue Element(queue=w415, timeout in ms (-1)=w409) -> (queue out=w418:refnum<queue>, element=w419:string)  [unwired: 1 in, 2 out]
    n171 = Match Pattern(string=w419, regular expression=":") -> (before substring=w417:string, after substring=w416:string)  [unwired: 1 in, 2 out]
    n172 = case shown="\"idle\", Default" w417 {
      tunnel: w418 -> [_ _ w436 w440 w449 w460]
      tunnel: w416 -> [_ _ _ _ _ _]
      tunnel: [_ _ _ _ TRUE _] -> w414
      tunnel: [w422 w424 w438 refnum<k5> refnum ("gateway_connection out") w447 w451] -> w413
      tunnel: [w421 w423 w437 w442 w446 w450] -> w412
      tunnel: w411 -> [w422 w424 w438 w444 w447 _]
      tunnel: w410 -> [w421 w423 w437 _ w446 _]
      tunnel: [_ _ -1 _ _ _] -> w408
      frame "idle", Default {
      }
      frame "relative" {
        n173 = disable-structure shown="Disabled" {
          frame Disabled {
            n174 = case shown="True" FALSE {
              tunnel: [_ w434] -> w426
              frame False {
              }
              frame True {
                n175 = call "sp_manip_get_axis_status.vi"("gateway_connection"=w434) -> ("error out"=w429:errorcluster, "axis_out"=w433:T5, "gateway_connection out"=w427:refnum<k5>)  [unwired: 6 in, 2 out]
                n176 = Index Array(array=w433) -> (element=w432:T6, index=w435:i32)
                n177 = Unbundle By Name(w432) -> ("Axis_Name"=w428:string)  [unwired: 1 out]
                n178 = Build Array(w428) -> (w431:string[])
                n179 = Build Array() -> (w430:void[])  [unwired: 1 in]
                n180 = call "sp_manip_start_move.vi"("error in"=w429, "target positions"=w430, "axis names"=w431, "gateway_connection"=w427) -> ()  [unwired: 4 in, 4 out]
              }
            }
          }
          frame Enabled {
          }
        }
      }
      frame "suspend" {
        n181 = Dequeue Element(queue=w436) -> ()  [unwired: 2 in, 4 out]
      }
      frame "release" {
        n182 = Dequeue Element(queue=w440) -> ()  [unwired: 2 in, 4 out]
        n183 = call "sp_manip_disconnect.vi"("gateway_connection"=w444) -> ("error out"=w443:errorcluster, "gateway_connection_out"=w445:refnum<k5>)  [unwired: 7 in, 2 out]
        n184 = call "tcp_gateway_close_connection.vi"("error in"=w443, "server_connection"=w445) -> ("error out"=w442:errorcluster)  [unwired: 5 in]
      }
      frame "close" {
        n185 = Release Queue(queue=w449) -> ()  [unwired: 2 in, 3 out]
      }
      frame "init" {
        n186 = Dequeue Element(queue=w460) -> ()  [unwired: 2 in, 4 out]
        n187 = call "tcp_gateway_open_connection.vi"() -> ("gateway_connection"=w455:refnum<k5>, "error out"=w454:errorcluster)  [unwired: 5 in, 3 out]
        n188 = call "sp_manip_connect.vi"("error in"=w454, "gateway_connection"=w455) -> ("error out"=w450:errorcluster, "axis_out"=w453:T5, "gateway_connection out"=w451:refnum<k5>)  [unwired: 5 in, 2 out]
        n189 = for {
          tunnel: w453 -> [w463] mode=indexing
          tunnel: [w462] -> w458 mode=indexing
          tunnel: [w461] -> w459 mode=indexing
          n190 = Unbundle By Name(w463) -> ("Axis_Name"=w462:string, "Axis_Position"=w461:dbl)
        }
        "names" <- w458
        "pos" <- w459
        n191 = control-ref of="meas_axis"() -> (w452:refnum<vi>)
        n192 = local write "dest"(w459) -> ()
        n193 = Build Array (concatenate)(w458, "XY") -> (w456:string[])
        n194 = property on="Property Node" class="CmbBox"(reference=w452, "Strings[]"=w456) -> ()  [unwired: 1 in, 2 out]
      }
    }
  }
  n195 = while {
    tunnel: w9 -> [w474]
    shift-right: [w471] -> _
    shift-left: 0 -> [w472]
    shift-right: [w470] -> _
    shift-left: _ -> [w469]
    shift-right: [w468] -> _
    shift-left: _ -> [w467]
    shift-right: [w466] -> _
    shift-left: u32 0 ("pHandle") -> [w465]
    tunnel: string[] ["Kinetic Energy", "Pass Energy", "Coil Current", "Work Function", "Detector Voltage", "Screen Voltage", "Conversion Voltage", "Focus Displacement 1", "Focus Displacement 2"] -> [w464]
    stop <- w473 stop-if-true
    n196 = Preview Queue Element(queue=w474, timeout in ms (-1)=w472) -> (queue out=w477:refnum<queue>, element=w478:string)  [unwired: 1 in, 2 out]
    n197 = Match Pattern(string=w478, regular expression=":") -> (before substring=w476:string, after substring=w475:string)  [unwired: 1 in, 2 out]
    n198 = case shown="\"idle\", Default" w476 {
      tunnel: w477 -> [_ w531 w547 w563 w577 w581 w587]
      tunnel: w475 -> [_ _ _ _ _ _ _]
      tunnel: [_ _ _ _ TRUE _ _] -> w473
      tunnel: [_ _ _ _ _ -1 _] -> w471
      tunnel: [w488 w533 w550 w561 w575 w580 w584] -> w470
      tunnel: w469 -> [w499 w522 w552 w562 w575 w580 _]
      tunnel: [w487 w532 w549 w560 w573 w578 w583] -> w468
      tunnel: w467 -> [w497 w521 w551 _ w573 w578 _]
      tunnel: [w485 w519 w548 w559 w574 w579 w586] -> w466
      tunnel: w465 -> [w485 w519 w548 w558 w574 w579 _]
      tunnel: w464 -> [w486 w512 _ _ _ _ _]
      frame "idle", Default {
        n199 = call "SL2_AD_DLL_Phoibos_GetDeviceState.vi"("dll_path"=w499, "pHandle_in"=w485, "dev_type"=DEF_dev_type."devA (analyzer)", "error in"=w497) -> ("path out"=w484:path, "state"=→"state":T1, "error out"=w483:errorcluster)  [unwired: 2 in]
        n200 = for {
          tunnel: w485 -> [w506]
          tunnel: w486 -> [w504] mode=indexing
          tunnel: [w503] -> w496 mode=indexing
          tunnel: [w502] -> w488
          shift-right: [w501] -> w487
          shift-left: w483 -> [w505]
          tunnel: w484 -> [w500]
          n201 = call "SL2_AD_DLL_Phoibos_GetVoltage.vi"("error in"=w505, "voltage_name"=w504, "pHandle"=w506, "dll path in"=w500) -> ("error out"=w501:errorcluster, "value"=w503:dbl, "dll path out"=w502:path)  [unwired: 3 in]
        }
        n202 = Index Array(array=w496) -> (element #1=→"phoib_I_1":dbl, element #2=→"phoib_I_2":dbl, element #3=→"phoib_I_3":dbl, element #4=→"phoib_I_4":dbl, element #5=→"phoib_I_5":dbl, element #6=→"phoib_I_6":dbl, element #7=→"phoib_I_7":dbl, element #8=→"phoib_I_8":dbl, element #9=→"phoib_I_9":dbl)  [unwired: 9 in]
      }
      frame "set" {
        n203 = Dequeue Element(queue=w531) -> ()  [unwired: 2 in, 4 out]
        n204 = Multiply(x="VoltageRange", y=13) -> (x*y=w528:i32)
        n205 = Add(x="Mode", y=w528) -> (x+y=w525:i32)
        n206 = Index Array(array=u32[] [251749632, 251749633, 251749634, 251749635, 251749636, 251749637, 251749638, 251749639, 251749640, 251749641, 251749642, 251749643, 251749644, 251749645, 251749646, 251749647, 251749648, 251749649, 251749650, 251749651, 251749652, 251749653, 251749654, 251749655, 251749656, 251749657, 251749658, 251749659, 251749660, 251749661, 251749662, 251749663, 251749664, 251749665, 251749666, 251749667, 251749668, 251749669, 251749670, 251749671, 251749672, 251749673, 251749674, 251749675, 251749676, 251749677, 251749678, 251749679, 251749680, 251749681, 251749682, 251749683, 251749684, 251749685, 251749686, 251749687, 251749688, 251749689, 251749690, 251749691, 251749692, 251749693, 251749694, 251749695, 251749696] ("modeIDs"), index=w525) -> (element=w523:u32)
        n207 = Build Array("phoib_I_1s", "phoib_I_2s", "phoib_I_3s", "phoib_I_4s", "phoib_I_5s", "phoib_I_6s", "phoib_I_7s", "phoib_I_8s", "phoib_I_9s") -> (w511:dbl[])
        n208 = call "SL2_AD_DLL_Phoibos_SetDeviceMode.vi"("pHandle"=w519, "error in"=w521, "value"=w523, "dev_type"=DEF_dev_type."devA (analyzer)", "dll path in"=w522) -> ("error out"=w510:errorcluster, "dll path out"=w520:path)  [unwired: 4 in]
        n209 = for {
          tunnel: w519 -> [w539]
          shift-right: [w546] -> w533
          shift-left: w520 -> [w543]
          tunnel: w512 -> [w538] mode=indexing
          tunnel: w511 -> [w537] mode=indexing
          shift-right: [w545] -> w532
          shift-left: w510 -> [w541]
          n210 = call "SL2_AD_DLL_Phoibos_GetVoltageRange.vi"("error in"=w541, "voltage_name"=w538, "pHandle"=w539, "dll path in"=w543) -> ("error out"=w540:errorcluster, "min"=w535:dbl, "max"=w536:dbl, "dll path out"=w542:path)  [unwired: 2 in]
          n211 = In Range and Coerce(upper limit=w536, x=w537, lower limit=w535) -> (coerced(x)=w534:dbl)  [unwired: 1 out]
          n212 = call "SL2_AD_DLL_Phoibos_SetVoltage.vi"("commit"=TRUE, "pHandle"=w539, "error in"=w540, "value"=w534, "voltageName"=w538, "dll path in"=w542) -> ("error out"=w545:errorcluster, "dll path out"=w546:path)  [unwired: 3 in]
        }
      }
      frame "standby" {
        w553 = T1 0 items=["Off"=-1, "Standby"=0, "On"=1] ("state")
        n213 = Dequeue Element(queue=w547) -> ()  [unwired: 2 in, 4 out]
        n214 = call "SL2_AD_DLL_Phoibos_SetDeviceState.vi"("pHandle_in"=w548, "error in"=w551, "state"=w553, "dev_type"=DEF_dev_type."devA (analyzer)", "dll_path"=w552) -> ("error out"=w549:errorcluster, "path out"=w550:path)  [unwired: 2 in]
      }
      frame "release" {
        n215 = Dequeue Element(queue=w563) -> ()  [unwired: 2 in, 4 out]
        n216 = flat-sequence {
          tunnel: w562 -> [w564]
          tunnel: w558 -> [w565]
          tunnel: [w568] -> w557
          tunnel: [w567] -> w556
          tunnel: [u32 0] -> w555
          tunnel: [w570] -> w559
          tunnel: [w571] -> w560
          tunnel: [w572] -> w561
          tunnel: w557 -> [w572]
          tunnel: w556 -> [w571]
          tunnel: w555 -> [w570]
          frame #0 {
            n217 = call "SL2_AD_DLL_Phoibos_Shutdown.vi"("pHandle"=w565, "dll path in"=w564) -> ("error out"=w567:errorcluster, "dll path out"=w568:path)  [unwired: 4 in]
          }
          frame #1 {
            n218 = local write "phoib_con?"(FALSE ("phoib_con?")) -> ()
          }
        }
      }
      frame "close" {
        n219 = Release Queue(queue=w577) -> ()  [unwired: 2 in, 3 out]
      }
      frame "suspend" {
        n220 = Dequeue Element(queue=w581) -> ()  [unwired: 2 in, 4 out]
      }
      frame "init" {
        n221 = Dequeue Element(queue=w587) -> ()  [unwired: 2 in, 4 out]
        n222 = flat-sequence {
          tunnel: [w594] -> w585
          tunnel: [w590] -> w584
          tunnel: [w589] -> w583
          tunnel: [w602] -> w586
          tunnel: w585 -> [w602]
          frame #0 {
            n223 = local write "phoib_con?"(FALSE ("phoib_con?")) -> ()
          }
          frame #1 {
            w593 = DEF_dev_type."devA (analyzer)" ("dev_type")
            n224 = call "GetSL2AD_VI_dllPath.vi"() -> ("error"=w597:errorcluster, "Path"=w598:path)  [unwired: 9 in, 1 out]
            n225 = call "SL2_AD_DLL_List_Devices.vi"("error in"=w597, "dev_type"=w593, "dll path in"=w598) -> ("error out"=w591:errorcluster, "devices"=w600:string[], "dll path out"=w592:path)  [unwired: 2 in]
            n226 = Index Array(array=w600) -> (element=w599:string)  [unwired: 1 in]
            n227 = call "SL2_AD_DLL_Phoibos_Initialize.vi"("error in"=w591, "analyzerId"=w599, "dll_path"=w592) -> ("error out"=w595:errorcluster, "pHandle"=w594:u32, "path out"=w596:path)  [unwired: 2 in]
            n228 = call "SL2_AD_DLL_Phoibos_ListDeviceModes.vi"("dll path in"=w596, "dev_type"=w593, "pHandle"=w594, "error in"=w595) -> ("dll path out"=w590:path, "error out"=w589:errorcluster)  [unwired: 1 in, 2 out]
          }
          frame #2 {
            n229 = local write "phoib_con?"(TRUE ("phoib_con?")) -> ()
          }
        }
      }
    }
    "error out 2" <- w468
  }
